vi "RSZVB Set Fixed Frequency.vi"(8 "error in (no error)":errorcluster {"code" format="%.0x"}, 9 "Fixed Frequency (300000.0 Hz)":dbl=300000.0 format="%^.3e", 10 "Channel (1)":i32=1, 11 "VISA session":refnum<visa-resource-name>) -> (0 "error out":errorcluster {"code" format="%.0x"}, 3 "dup VISA session":refnum<visa-resource-name>)   [LabVIEW 2011]
doc: "This VI defines a fixed frequency, to be assigned either to the RF, the LO, or the IF signal.\n\nRemote-control command(s):\n[SENSe<Ch>:]FREQuency:CONVersion:MIXer:FFIXed <fixed_frequency>"
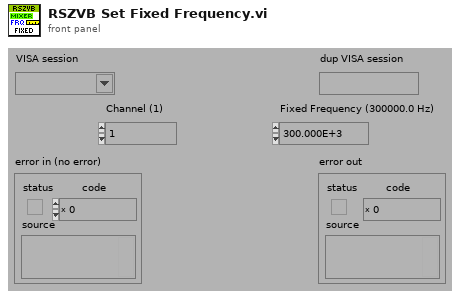
[diagram p1: front panel]
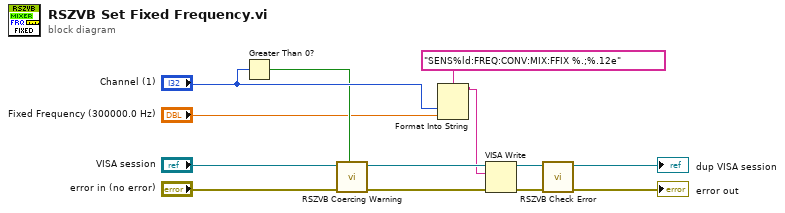
[diagram p0: block diagram]
diagram:
  n1 = Greater Than 0?(x="Channel (1)") -> (x > 0?=w2:bool)
  n2 = call "RSZVB Coercing Warning.vi"("In Range?"=w2, "error in (no error)"="error in (no error)", "VISA session"="VISA session") -> ("error out"=w12:errorcluster, "dup VISA session"=w13:refnum<visa-resource-name>)  [unwired: 7 in]
  n3 = Format Into String(format string="SENS%ld:FREQ:CONV:MIX:FFIX %.;%.12e", "Channel (1)", "Fixed Frequency (300000.0 Hz)") -> (resulting string=w8:string)  [unwired: 2 in, 1 out]
  n4 = VISA Write(VISA resource name=w13, write buffer=w8, error in (no error)=w12) -> (VISA resource name out=w10:refnum<visa-resource-name>, error out=w11:errorcluster)  [unwired: 1 out]
  n5 = call "RSZVB Check Error.vi"("error in (no error)"=w11, "VISA session"=w10) -> ("error out"=→"error out":errorcluster, "dup VISA session"=→"dup VISA session":refnum<visa-resource-name>)  [unwired: 8 in]
